vi "SetMatrixExperiment.vi"() -> ()   [LabVIEW 2014]
uses:
  <vilib>/Utility/file.llb/Write To Spreadsheet File (I64).vi
panel:
  out "Large Array":bool[][][](array[boolean])
  out "Configuration file:":path
  in  "Save end Exit":bool
  in  "Enter total number of\ncontact configurations\nto be measured":i8=3
  in  "Choose configuration # and manually \nenter connections on the right table.":u16(ring) items=["Configuration #1", "Configuration #2"]
  in  "Table":bool[][](array[boolean])
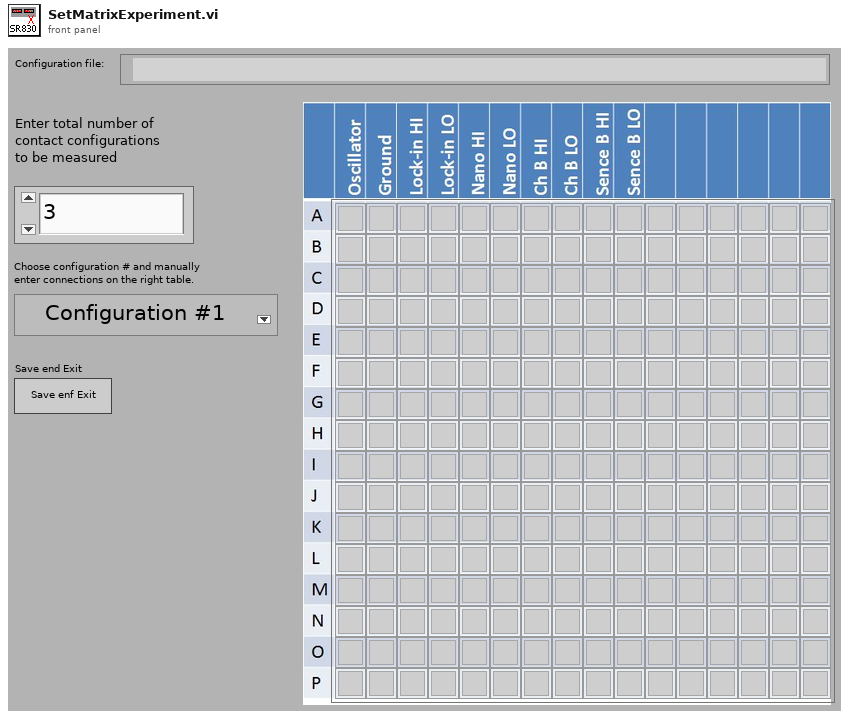
[diagram p1: front panel]
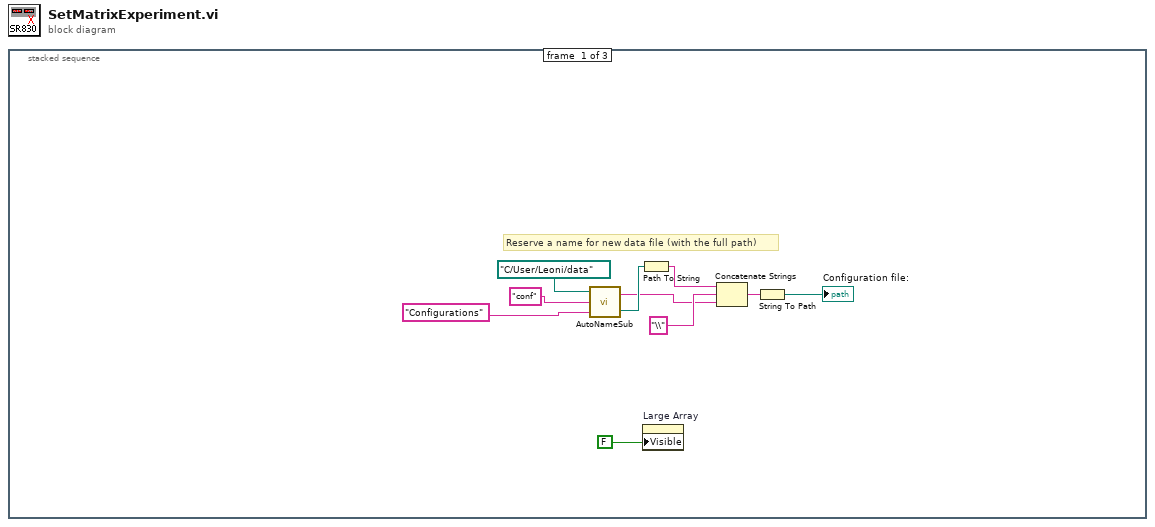
[diagram p0: block diagram]
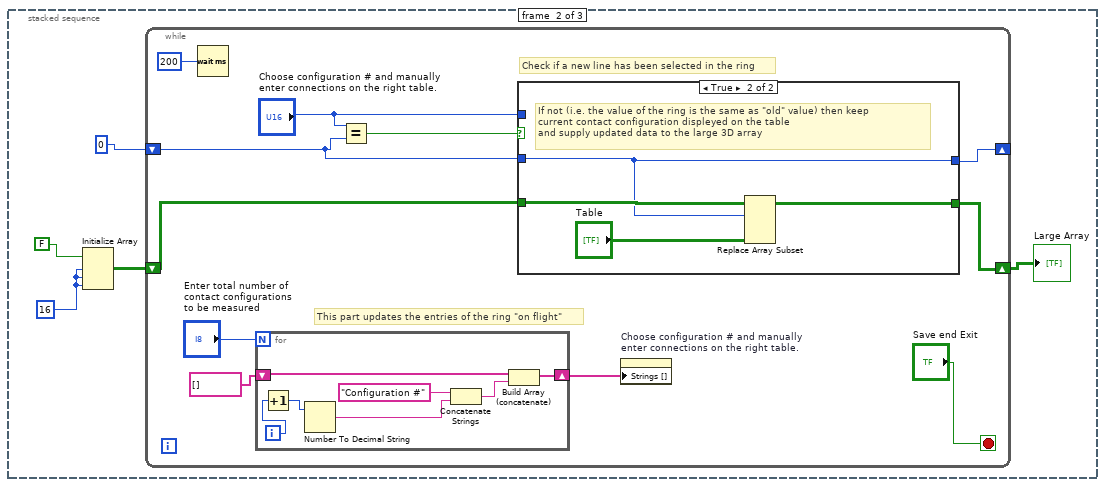
[diagram p2: hidden frame]
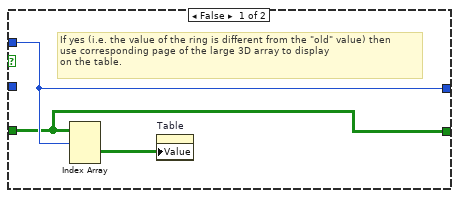
[diagram p3: hidden frame]
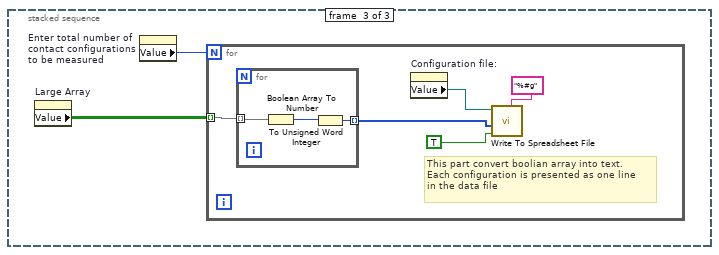
[diagram p4: hidden frame]
diagram:
  n1 = stacked-sequence {
    frame #0 {
      # "Reserve a name for new data file (with the full path)"
      n2 = call "AutoNameSub.vi"("Custom Folder"="Configurations", "Extention"="conf", "User Data Folder"=path "C:/User/Leoni/data") -> ("created path"=w5:path, "String"=w4:string)
      n3 = Path To String(path=w5) -> (string=w10:string)
      n4 = property on="Large Array" class="Arr (strict)"("Visible"=FALSE) -> ()  [unwired: 2 in, 2 out]
      n5 = Concatenate Strings(w10, "\\", w4) -> (w8:string)
      n6 = String To Path(string=w8) -> (path=→"Configuration file:":path)
    }
    frame #1 {
      w12 = 16
      n7 = Initialize Array(FALSE, w12, w12, w12) -> (w13:bool[][][])
      n8 = while {
        shift-right: [w19] -> _
        shift-left: 0 -> [w21]
        shift-right: [w16] -> w11
        shift-left: w13 -> [w17]
        stop <- "Save end Exit" stop-if-true
        # "This part updates the entries of the ring \"on flight\""
        # "Check if a new line has been selected in the ring"
        n9 = Wait (ms)(milliseconds to wait=200) -> ()  [unwired: 1 out]
        n10 = for {
          N: "Enter total number of\ncontact configurations\nto be measured" -> [_]
          shift-right: [w37] -> w25
          shift-left: string[] [] -> [w38]
          i -> [w35]
          n11 = Increment(x=w35) -> (x+1=w34:i32)
          n12 = Number To Decimal String(number=w34) -> (decimal integer string=w39:string)  [unwired: 1 in]
          n13 = Concatenate Strings("Configuration #", w39) -> (w36:string)
          n14 = Build Array (concatenate)(w38, w36) -> (w37:string[])
        }
        n15 = Equal?(x="Choose configuration # and manually \nenter connections on the right table.", y=w21) -> (x = y?=w22:bool)
        n16 = case shown="True" w22 {
          tunnel: "Choose configuration # and manually \nenter connections on the right table." -> [w29 _]
          tunnel: w21 -> [_ w30]
          tunnel: [w29 w30] -> w19
          tunnel: w17 -> [w27 w33]
          tunnel: [w27 w31] -> w16
          frame False {
            # "If yes (i.e. the value of the ring is different from the \"old\" value) then \nuse corresponding page of the large 3D array to display\non the table."
            n17 = Index Array(array=w27, index (dim 0)=w29) -> (element=w28:bool[][])  [unwired: 2 in]
            n18 = property on="Table" class="Arr (strict)"("Value"=w28) -> ()  [unwired: 2 in, 2 out]
          }
          frame True {
            # "If not (i.e. the value of the ring is the same as \"old\" value) then keep \ncurrent contact configuration displeyed on the table\nand supply updated data to the large 3D array"
            n19 = Replace Array Subset(array=w33, new element="Table", index (dim 0)=w30) -> (w31:bool[][][])  [unwired: 2 in]
          }
        }
        n20 = property on="Choose configuration # and manually \nenter connections on the right table." class="Ring (strict)"("Strings []"=w25) -> ()  [unwired: 2 in, 2 out]
      }
      "Large Array" <- w11
    }
    frame #2 {
      n21 = property on="Large Array" class="Arr (strict)"() -> ("Value"=w41:bool[][][])  [unwired: 2 in, 2 out]
      n22 = property on="Enter total number of\ncontact configurations\nto be measured" class="DigNum (strict)"() -> ("Value"=w42:i8)  [unwired: 2 in, 2 out]
      n23 = for {
        N: w42 -> [_]
        tunnel: w41 -> [w43] mode=indexing
        # "This part convert boolian array into text. \nEach configuration is presented as one line \nin the data file"
        n24 = for {
          tunnel: [w49] -> w45 mode=indexing
          tunnel: w43 -> [w48] mode=indexing
          n25 = Boolean Array To Number(Boolean array=w48) -> (number=w50:u32)
          n26 = To Unsigned Word Integer(number=w50) -> (unsigned 16bit integer=w49:u16)
        }
        n27 = property on="Configuration file:" class="Path"() -> ("Value"=w44:path)  [unwired: 2 in, 2 out]
        n28 = call-poly <vilib>:"Write To Spreadsheet File.vi"("format (%d)"="%#g", "append to file? (new file:F)"=TRUE, "1D data"=w45, "file path (dialog if empty)"=w44) -> ()  [unwired: 4 in, 1 out]
      }
    }
  }
